vi "16-ParseContent.vi"(10 "TypeID":T1(ring), 11 "BITS in":bool[](array[boolean])) -> (2 "Content":variant, 3 "BITS out":bool[](array[boolean]))   [LabVIEW 2019, in "16.lvlib"]
uses:
  16.lvlib
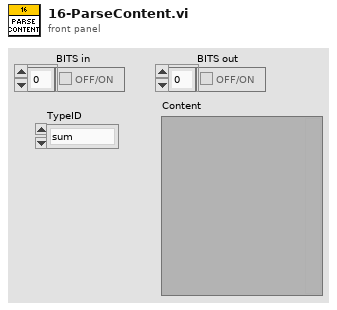
[diagram p1: front panel]
types:
  T1 = enum16{"sum", "product", "minimum", "maximum", "literal", "greater than", "less than", "equal to"}
  T2 = cluster{"Version":u32, "TypeID":enum16{"sum", "product", "minimum", "maximum", "literal", "greater than", "less than", "equal to"}, "Content":variant}[]
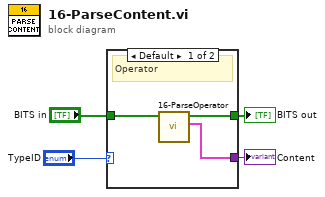
[diagram p0: block diagram]
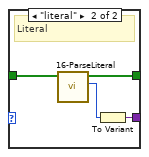
[diagram p2: hidden frame]
diagram:
  n1 = case shown="Default" "TypeID" {
    tunnel: "BITS in" -> [w6 w11]
    tunnel: [w7 w9] -> w3
    tunnel: [w5 w8] -> w1
    frame Default {
      # "Operator"
      n2 = call "16-ParseOperator.vi"("BITS in"=w6) -> ("Packets"=w5:T2, "BITS out"=w7:bool[])  [unwired: 9 in]
    }
    frame "literal" {
      # "Literal"
      n3 = call "16-ParseLiteral.vi"("BITS in"=w11) -> ("Value"=w10:u64, "BITS out"=w9:bool[])  [unwired: 9 in]
      n4 = To Variant(anything=w10) -> (Variant=w8:variant)
    }
  }
  "BITS out" <- w3
  "Content" <- w1
